vi "FTW-CodeGen-FindTerm.vi"(5 "Terms":T2(array[cluster]), 7 "Terminal ID":string) -> (4 "Index":i32, 6 "Term":T1, 8 "Found?":bool)   [LabVIEW 2015]
panel:
  # "Inputs"
  # "Outputs"
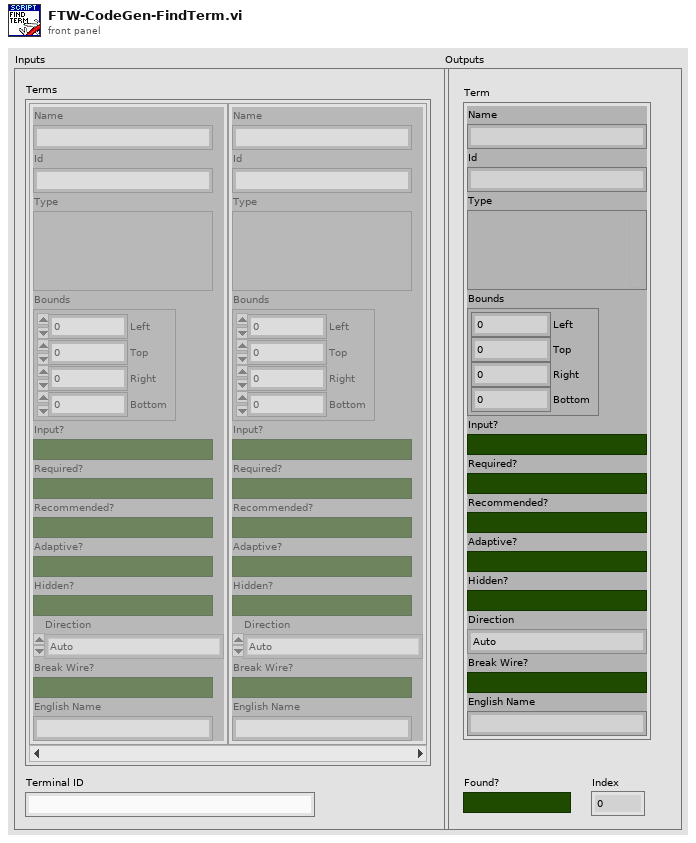
[diagram p1: front panel]
types:
  T1 = cluster{"Name":string, "Id":string, "Type":variant, "Bounds":cluster{"Left":i32, "Top":i32, "Right":i32, "Bottom":i32}, "Input?":bool, "Required?":bool, "Recommended?":bool, "Adaptive?":bool, "Hidden?":bool, "Direction":enum32{"Auto", "Up", "Down", "Left", "Right", "Center"}, "Break Wire?":bool, "English Name":string}
  T2 = cluster{"Name":string, "Id":string, "Type":variant, "Bounds":cluster{"Left":i32, "Top":i32, "Right":i32, "Bottom":i32}, "Input?":bool, "Required?":bool, "Recommended?":bool, "Adaptive?":bool, "Hidden?":bool, "Direction":enum32{"Auto", "Up", "Down", "Left", "Right", "Center"}, "Break Wire?":bool, "English Name":string}[]
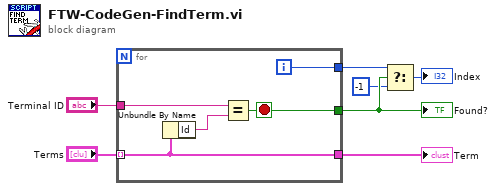
[diagram p0: block diagram]
diagram:
  n1 = for {
    tunnel: [w9] -> w6
    tunnel: [w12] -> w4
    tunnel: "Terms" -> [w9] mode=indexing
    tunnel: "Terminal ID" -> [w10]
    tunnel: [w8] -> w3
    i -> [w8]
    stop <- w12 stop-if-true
    n2 = Unbundle By Name(w9) -> ("Id"=w11:string)
    n3 = Equal?(x=w10, y=w11) -> (x = y?=w12:bool)
  }
  "Term" <- w6
  "Found?" <- w4
  n4 = Select(t=w3, s=w4, f=-1) -> (s? t:f=→"Index":i32)
